vi "+S2C_Shared_Function.vi"(8 "Error In":errorcluster, 11 "Settings":T1) -> (0 "Error Out":errorcluster, 3 "Response":string)   [LabVIEW 2015]
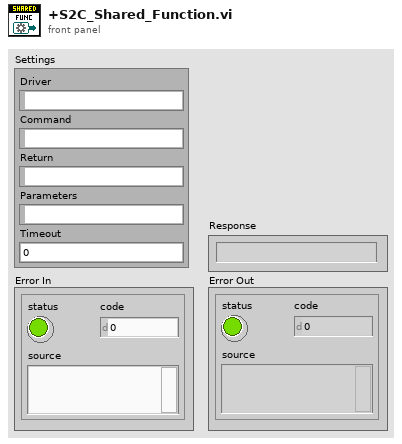
[diagram p1: front panel]
types:
  T1 = cluster{"Driver":string, "Command":string, "Return":string, "Parameters":string, "Timeout":dbl}
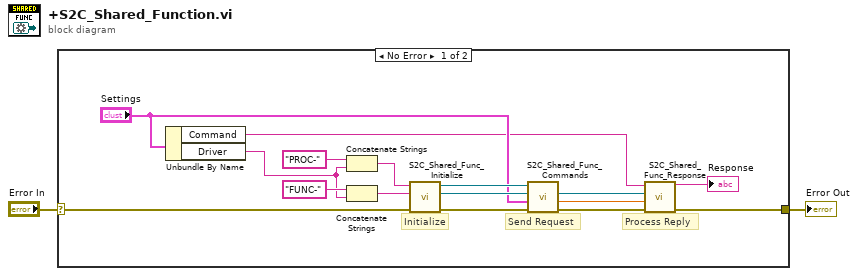
[diagram p0: block diagram]
diagram:
  n1 = case shown="No Error" "Error In" {
    selector: "Error In" -> [w18 w19]
    tunnel: [w17 w19] -> w1
    frame No Error {
      # "Send Request"
      # "Process Reply"
      # "Initialize"
      n2 = Unbundle By Name("Settings") -> ("Command"=w3:string, "Driver"=w4:string)
      n3 = Concatenate Strings("PROC-" ("string"), w4) -> (w7:string)
      n4 = Concatenate Strings("FUNC-" ("string"), w4) -> (w8:string)
      n5 = call "S2C_Shared_Func_Initialize.vi"("Error In"=w18, "Func-Q-Name"=w8, "Cmd-Q-Name"=w7) -> ("Error Out"=w12:errorcluster, "Func-Q"=w13:refnum<queue>, "Cmd-Q"=w14:refnum<queue>)  [unwired: 6 in]
      n6 = call "S2C_Shared_Func_Commands.vi"("Error In"=w12, "Settings"="Settings", "Func-Q In"=w13, "Proc-Q"=w14) -> ("Error Out"=w16:errorcluster, "Timeout"=w15:dbl, "Func-Q Out"=w6:refnum<queue>)  [unwired: 5 in]
      n7 = call "S2C_Shared_Func_Response.vi"("Error In"=w16, "Timeout"=w15, "Func-Q"=w6, "Command"=w3) -> ("Error Out"=w17:errorcluster, "Response"=→"Response":string)  [unwired: 6 in]
    }
    frame Error {
    }
  }
  "Error Out" <- w1
